vi "Methods_Insert Dividers.vi"(11 "Methods[] In":T1(array[cluster])) -> (3 "Methods[] Out":T1(array[cluster]))   [LabVIEW 2023] (continued)
, "Class Name (unlocalized)"="EventStructure", "Class Name (localized)"="EventStructure"}, "Method Info"={"Unique ID string"="5191803", "Data name"="SetHandledEvents", "Short name (localized)"="SetHandledEvents", "Long name (localized)"="Set Handled Events"}, "Method Flags"={"IsDeprecated"=FALSE, "IsPrivate"=FALSE, "IsScripting"=TRUE, "IsNotInRun-Time"=TRUE}, "Divider"=FALSE}, {"Class Info"={"Unique ID string"="16458", "Parent ID string"="16406", "Class Name (unlocalized)"="EventStructure", "Class Name (localized)"="EventStructure"}, "Method Info"={"Unique ID string"="5191804", "Data name"="GetHandledEventsPriv", "Short name (localized)"="GetHandledEventsPriv", "Long name (localized)"="Get Handled Events (Private)"}, "Method Flags"={"IsDeprecated"=FALSE, "IsPrivate"=TRUE, "IsScripting"=TRUE, "IsNotInRun-Time"=TRUE}, "Divider"=FALSE}, {"Class Info"={"Unique ID string"="16458", "Parent ID string"="16406", "Class Name (unlocalized)"="EventStructure", "Class Name (localized)"="EventStructure"}, "Method Info"={"Unique ID string"="5191805", "Data name"="SetHandledEventsPriv", "Short name (localized)"="SetHandledEventsPriv", "Long name (localized)"="Set Handled Events (Private)"}, "Method Flags"={"IsDeprecated"=FALSE, "IsPrivate"=TRUE, "IsScripting"=TRUE, "IsNotInRun-Time"=TRUE}, "Divider"=FALSE}, {"Class Info"={"Unique ID string"="16459", "Parent ID string"="36", "Class Name (unlocalized)"="FlatSequence", "Class Name (localized)"="FlatSequence"}, "Method Info"={"Unique ID string"="3578b800", "Data name"="Add Frame", "Short name (localized)"="Add Frame", "Long name (localized)"="Add Frame"}, "Method Flags"={"IsDeprecated"=FALSE, "IsPrivate"=FALSE, "IsScripting"=TRUE, "IsNotInRun-Time"=FALSE}, "Divider"=FALSE}, {"Class Info"={"Unique ID string"="16459", "Parent ID string"="36", "Class Name (unlocalized)"="FlatSequence", "Class Name (localized)"="FlatSequence"}, "Method Info"={"Unique ID string"="3578b801", "Data name"="Remove Frame", "Short name (localized)"="Remove Frame", "Long name (localized)"="Remove Frame"}, "Method Flags"={"IsDeprecated"=FALSE, "IsPrivate"=FALSE, "IsScripting"=TRUE, "IsNotInRun-Time"=FALSE}, "Divider"=FALSE}, {"Class Info"={"Unique ID string"="16459", "Parent ID string"="36", "Class Name (unlocalized)"="FlatSequence", "Class Name (localized)"="FlatSequence"}, "Method Info"={"Unique ID string"="3578b802", "Data name"="Auto Size", "Short name (localized)"="Auto Size", "Long name (localized)"="Auto Size"}, "Method Flags"={"IsDeprecated"=FALSE, "IsPrivate"=FALSE, "IsScripting"=TRUE, "IsNotInRun-Time"=FALSE}, "Divider"=FALSE}, {"Class Info"={"Unique ID string"="16459", "Parent ID string"="36", "Class Name (unlocalized)"="FlatSequence", "Class Name (localized)"="FlatSequence"}, "Method Info"={"Unique ID string"="3578b803", "Data name"="Remove Flat Sequence", "Short name (localized)"="Remove Flat Sequence", "Long name (localized)"="Remove Flat Sequence"}, "Method Flags"={"IsDeprecated"=FALSE, "IsPrivate"=FALSE, "IsScripting"=TRUE, "IsNotInRun-Time"=FALSE}, "Divider"=FALSE}, {"Class Info"={"Unique ID string"="16459", "Parent ID string"="36", "Class Name (unlocalized)"="FlatSequence", "Class Name (localized)"="FlatSequence"}, "Method Info"={"Unique ID string"="3578b805", "Data name"="Convert To TimedSequence", "Short name (localized)"="Convert To TimedSequence", "Long name (localized)"="Convert To Timed Sequence"}, "Method Flags"={"IsDeprecated"=FALSE, "IsPrivate"=FALSE, "IsScripting"=TRUE, "IsNotInRun-Time"=FALSE}, "Divider"=FALSE}, {"Class Info"={"Unique ID string"="16463", "Parent ID string"="3", "Class Name (unlocalized)"="SubWizard", "Class Name (localized)"="SubWizard"}, "Method Info"={"Unique ID string"="31942800", "Data name"="LockObject", "Short name (localized)"="LockObject", "Long name (localized)"="Lock Object"}, "Method Flags"={"IsDeprecated"=FALSE, "IsPrivate"=FALSE, "IsScripting"=TRUE, "IsNotInRun-Time"=FALSE}, "Divider"=FALSE}, {"Class Info"={"Unique ID string"="16463", "Parent ID string"="3", "Class Name (unlocalized)"="SubWizard", "Class Name (localized)"="SubWizard"}, "Method Info"={"Unique ID string"="31942801", "Data name"="UnLock Object", "Short name (localized)"="UnLock Object", "Long name (localized)"="Unlock Object"}, "Method Flags"={"IsDeprecated"=FALSE, "IsPrivate"=FALSE, "IsScripting"=TRUE, "IsNotInRun-Time"=FALSE}, "Divider"=FALSE}, {"Class Info"={"Unique ID string"="16463", "Parent ID string"="3", "Class Name (unlocalized)"="SubWizard", "Class Name (localized)"="SubWizard"}, "Method Info"={"Unique ID string"="31942802", "Data name"="Is Locked By Me", "Short name (localized)"="Is Locked By Me", "Long name (localized)"="Is Locked By Me"}, "Method Flags"={"IsDeprecated"=FALSE, "IsPrivate"=FALSE, "IsScripting"=TRUE, "IsNotInRun-Time"=FALSE}, "Divider"=FALSE}, {"Class Info"={"Unique ID string"="16463", "Parent ID string"="3", "Class Name (unlocalized)"="SubWizard", "Class Name (localized)"="SubWizard"}, "Method Info"={"Unique ID string"="31942803", "Data name"="Lock Const", "Short name (localized)"="Lock Const", "Long name (localized)"="Lock Const"}, "Method Flags"={"IsDeprecated"=FALSE, "IsPrivate"=FALSE, "IsScripting"=TRUE, "IsNotInRun-Time"=FALSE}, "Divider"=FALSE}, {"Class Info"={"Unique ID string"="16463", "Parent ID string"="3", "Class Name (unlocalized)"="SubWizard", "Class Name (localized)"="SubWizard"}, "Method Info"={"Unique ID string"="31942804", "Data name"="UnLock Const", "Short name (localized)"="UnLock Const", "Long name (localized)"="Unlock Const"}, "Method Flags"={"IsDeprecated"=FALSE, "IsPrivate"=FALSE, "IsScripting"=TRUE, "IsNotInRun-Time"=FALSE}, "Divider"=FALSE}, {"Class Info"={"Unique ID string"="16467", "Parent ID string"="16435", "Class Name (unlocalized)"="TimedLoop", "Class Name (localized)"="TimedLoop"}, "Method Info"={"Unique ID string"="5afcf000", "Data name"="Replace With WhileLoop", "Short name (localized)"="Replace With WhileLoop", "Long name (localized)"="Replace With WhileLoop"}, "Method Flags"={"IsDeprecated"=FALSE, "IsPrivate"=FALSE, "IsScripting"=TRUE, "IsNotInRun-Time"=FALSE}, "Divider"=FALSE}, {"Class Info"={"Unique ID string"="16467", "Parent ID string"="16435", "Class Name (unlocalized)"="TimedLoop", "Class Name (localized)"="TimedLoop"}, "Method Info"={"Unique ID string"="5afcf001", "Data name"="Replace With TimedSeq", "Short name (localized)"="Replace With TimedSeq", "Long name (localized)"="Replace With TimedSequence"}, "Method Flags"={"IsDeprecated"=FALSE, "IsPrivate"=FALSE, "IsScripting"=TRUE, "IsNotInRun-Time"=FALSE}, "Divider"=FALSE}, {"Class Info"={"Unique ID string"="16472", "Parent ID string"="16384", "Class Name (unlocalized)"="SimDiagram", "Class Name (localized)"="SimDiagram"}, "Method Info"={"Unique ID string"="790ac00", "Data name"="CopyToCompanion", "Short name (localized)"="CopyToCompanion", "Long name (localized)"="CopyToCompanion"}, "Method Flags"={"IsDeprecated"=FALSE, "IsPrivate"=TRUE, "IsScripting"=TRUE, "IsNotInRun-Time"=FALSE}, "Divider"=FALSE}, {"Class Info"={"Unique ID string"="16472", "Parent ID string"="16384", "Class Name (unlocalized)"="SimDiagram", "Class Name (localized)"="SimDiagram"}, "Method Info"={"Unique ID string"="790ac01", "Data name"="setNodeMap", "Short name (localized)"="setNodeMap", "Long name (localized)"="setNodeMap"}, "Method Flags"={"IsDeprecated"=FALSE, "IsPrivate"=TRUE, "IsScripting"=TRUE, "IsNotInRun-Time"=FALSE}, "Divider"=FALSE}, {"Class Info"={"Unique ID string"="16472", "Parent ID string"="16384", "Class Name (unlocalized)"="SimDiagram", "Class Name (localized)"="SimDiagram"}, "Method Info"={"Unique ID string"="790ac02", "Data name"="setSignalMap", "Short name (localized)"="setSignalMap", "Long name (localized)"="setSignalMap"}, "Method Flags"={"IsDeprecated"=FALSE, "IsPrivate"=TRUE, "IsScripting"=TRUE, "IsNotInRun-Time"=FALSE}, "Divider"=FALSE}, {"Class Info"={"Unique ID string"="16472", "Parent ID string"="16384", "Class Name (unlocalized)"="SimDiagram", "Class Name (localized)"="SimDiagram"}, "Method Info"={"Unique ID string"="790ac03", "Data name"="SubsystemFromSelection", "Short name (localized)"="SubsystemFromSelection", "Long name (localized)"="Subsystem From Selection"}, "Method Flags"={"IsDeprecated"=FALSE, "IsPrivate"=TRUE, "IsScripting"=TRUE, "IsNotInRun-Time"=FALSE}, "Divider"=FALSE}, {"Class Info"={"Unique ID string"="16473", "Parent ID string"="16384", "Class Name (unlocalized)"="CompanionDiagram", "Class Name (localized)"="CompanionDiagram"}, "Method Info"={"Unique ID string"="7684bc00", "Data name"="SplitCaseStruct", "Short name (localized)"="SplitCaseStruct", "Long name (localized)"="SplitCaseStruct"}, "Method Flags"={"IsDeprecated"=FALSE, "IsPrivate"=TRUE, "IsScripting"=TRUE, "IsNotInRun-Time"=TRUE}, "Divider"=FALSE}, {"Class Info"={"Unique ID string"="16476", "Parent ID string"="16410", "Class Name (unlocalized)"="Bundler", "Class Name (localized)"="Bundler"}, "Method Info"={"Unique ID string"="570ad000", "Data name"="AddInputAfter", "Short name (localized)"="AddInputAfter", "Long name (localized)"="AddInputAfter"}, "Method Flags"={"IsDeprecated"=FALSE, "IsPrivate"=FALSE, "IsScripting"=TRUE, "IsNotInRun-Time"=TRUE}, "Divider"=FALSE}, {"Class Info"={"Unique ID string"="16476", "Parent ID string"="16410", "Class Name (unlocalized)"="Bundler", "Class Name (localized)"="Bundler"}, "Method Info"={"Unique ID string"="570ad001", "Data name"="RemoveInput", "Short name (localized)"="RemoveInput", "Long name (localized)"="RemoveInput"}, "Method Flags"={"IsDeprecated"=FALSE, "IsPrivate"=FALSE, "IsScripting"=TRUE, "IsNotInRun-Time"=TRUE}, "Divider"=FALSE}, {"Class Info"={"Unique ID string"="16477", "Parent ID string"="16410", "Class Name (unlocalized)"="Unbundler", "Class Name (localized)"="Unbundler"}, "Method Info"={"Unique ID string"="5cc5a000", "Data name"="AddOutputAfter", "Short name (localized)"="AddOutputAfter", "Long name (localized)"="Add Output After"}, "Method Flags"={"IsDeprecated"=FALSE, "IsPrivate"=FALSE, "IsScripting"=TRUE, "IsNotInRun-Time"=TRUE}, "Divider"=FALSE}, {"Class Info"={"Unique ID string"="16477", "Parent ID string"="16410", "Class Name (unlocalized)"="Unbundler", "Class Name (localized)"="Unbundler"}, "Method Info"={"Unique ID string"="5cc5a001", "Data name"="RemoveOutput", "Short name (localized)"="RemoveOutput", "Long name (localized)"="Remove Output"}, "Method Flags"={"IsDeprecated"=FALSE, "IsPrivate"=FALSE, "IsScripting"=TRUE, "IsNotInRun-Time"=TRUE}, "Divider"=FALSE}, {"Class Info"={"Unique ID string"="16485", "Parent ID string"="16421", "Class Name (unlocalized)"="XNode", "Class Name (localized)"="XNode"}, "Method Info"={"Unique ID string"="5f11b402", "Data name"="Message", "Short name (localized)"="Message", "Long name (localized)"="Message"}, "Method Flags"={"IsDeprecated"=FALSE, "IsPrivate"=TRUE, "IsScripting"=TRUE, "IsNotInRun-Time"=TRUE}, "Divider"=FALSE}, {"Class Info"={"Unique ID string"="16485", "Parent ID string"="16421", "Class Name (unlocalized)"="XNode", "Class Name (localized)"="XNode"}, "Method Info"={"Unique ID string"="5f11b403", "Data name"="AddLinkerReference", "Short name (localized)"="AddLinkerReference", "Long name (localized)"="AddLinkerReference"}, "Method Flags"={"IsDeprecated"=FALSE, "IsPrivate"=TRUE, "IsScripting"=TRUE, "IsNotInRun-Time"=TRUE}, "Divider"=FALSE}, {"Class Info"={"Unique ID string"="16485", "Parent ID string"="16421", "Class Name (unlocalized)"="XNode", "Class Name (localized)"="XNode"}, "Method Info"={"Unique ID string"="5f11b404", "Data name"="GetLinkerReference", "Short name (localized)"="GetLinkerReference", "Long name (localized)"="GetLinkerReference"}, "Method Flags"={"IsDeprecated"=FALSE, "IsPrivate"=TRUE, "IsScripting"=TRUE, "IsNotInRun-Time"=TRUE}, "Divider"=FALSE}, {"Class Info"={"Unique ID string"="16485", "Parent ID string"="16421", "Class Name (unlocalized)"="XNode", "Class Name (localized)"="XNode"}, "Method Info"={"Unique ID string"="5f11b405", "Data name"="RemoveLinkerReference", "Short name (localized)"="RemoveLinkerReference", "Long name (localized)"="Remove Linker Reference"}, "Method Flags"={"IsDeprecated"=FALSE, "IsPrivate"=TRUE, "IsScripting"=TRUE, "IsNotInRun-Time"=TRUE}, "Divider"=FALSE}, {"Class Info"={"Unique ID string"="16485", "Parent ID string"="16421", "Class Name (unlocalized)"="XNode", "Class Name (localized)"="XNode"}, "Method Info"={"Unique ID string"="5f11b406", "Data name"="RemoveXNode", "Short name (localized)"="RemoveXNode", "Long name (localized)"="Remove XNode"}, "Method Flags"={"IsDeprecated"=FALSE, "IsPrivate"=TRUE, "IsScripting"=TRUE, "IsNotInRun-Time"=FALSE}, "Divider"=FALSE}, {"Class Info"={"Unique ID string"="16485", "Parent ID string"="16421", "Class Name (unlocalized)"="XNode", "Class Name (localized)"="XNode"}, "Method Info"={"Unique ID string"="5f11b407", "Data name"="GetOtherTerminal", "Short name (localized)"="GetOtherTerminal", "Long name (localized)"="Get Other Terminal"}, "Method Flags"={"IsDeprecated"=FALSE, "IsPrivate"=TRUE, "IsScripting"=TRUE, "IsNotInRun-Time"=FALSE}, "Divider"=FALSE}, {"Class Info"={"Unique ID string"="16485", "Parent ID string"="16421", "Class Name (unlocalized)"="XNode", "Class Name (localized)"="XNode"}, "Method Info"={"Unique ID string"="5f11b408", "Data name"="GenerateCode", "Short name (localized)"="GenerateCode", "Long name (localized)"="Generate Code"}, "Method Flags"={"IsDeprecated"=FALSE, "IsPrivate"=TRUE, "IsScripting"=TRUE, "IsNotInRun-Time"=TRUE}, "Divider"=FALSE}, {"Class Info"={"Unique ID string"="16485", "Parent ID string"="16421", "Class Name (unlocalized)"="XNode", "Class Name (localized)"="XNode"}, "Method Info"={"Unique ID string"="5f11b40a", "Data name"="GetTermByID", "Short name (localized)"="GetTermByID", "Long name (localized)"="Get Term By ID"}, "Method Flags"={"IsDeprecated"=FALSE, "IsPrivate"=TRUE, "IsScripting"=TRUE, "IsNotInRun-Time"=FALSE}, "Divider"=FALSE}, {"Class Info"={"Unique ID string"="16485", "Parent ID string"="16421", "Class Name (unlocalized)"="XNode", "Class Name (localized)"="XNode"}, "Method Info"={"Unique ID string"="5f11b40b", "Data name"="XSFP.Set Terms", "Short name (localized)"="XSFP.Set Terms", "Long name (localized)"="XSFP:Set Terminals"}, "Method Flags"={"IsDeprecated"=FALSE, "IsPrivate"=TRUE, "IsScripting"=TRUE, "IsNotInRun-Time"=FALSE}, "Divider"=FALSE}, {"Class Info"={"Unique ID string"="16485", "Parent ID string"="16421", "Class Name (unlocalized)"="XNode", "Class Name (localized)"="XNode"}, "Method Info"={"Unique ID string"="5f11b40c", "Data name"="XSFP.SetBounds", "Short name (localized)"="XSFP.SetBounds", "Long name (localized)"="XSFP:Set Bounds"}, "Method Flags"={"IsDeprecated"=FALSE, "IsPrivate"=TRUE, "IsScripting"=TRUE, "IsNotInRun-Time"=FALSE}, "Divider"=FALSE}, {"Class Info"={"Unique ID string"="16485", "Parent ID string"="16421", "Class Name (unlocalized)"="XNode", "Class Name (localized)"="XNode"}, "Method Info"={"Unique ID string"="5f11b40d", "Data name"="SelectMenuNoReply", "Short name (localized)"="SelectMenuNoReply", "Long name (localized)"="SelectMenu No Reply"}, "Method Flags"={"IsDeprecated"=FALSE, "IsPrivate"=TRUE, "IsScripting"=TRUE, "IsNotInRun-Time"=FALSE}, "Divider"=FALSE}, {"Class Info"={"Unique ID string"="16485", "Parent ID string"="16421", "Class Name (unlocalized)"="XNode", "Class Name (localized)"="XNode"}, "Method Info"={"Unique ID string"="5f11b40e", "Data name"="ValueForTerm", "Short name (localized)"="ValueForTerm", "Long name (localized)"="ValueForTerm"}, "Method Flags"={"IsDeprecated"=FALSE, "IsPrivate"=TRUE, "IsScripting"=TRUE, "IsNotInRun-Time"=TRUE}, "Divider"=FALSE}, {"Class Info"={"Unique ID string"="16485", "Parent ID string"="16421", "Class Name (unlocalized)"="XNode", "Class Name (localized)"="XNode"}, "Method Info"={"Unique ID string"="5f11b40f", "Data name"="XSFP.Clear Diagram", "Short name (localized)"="XSFP.Clear Diagram", "Long name (localized)"="XSFP:Clear"}, "Method Flags"={"IsDeprecated"=FALSE, "IsPrivate"=TRUE, "IsScripting"=TRUE, "IsNotInRun-Time"=FALSE}, "Divider"=FALSE}, {"Class Info"={"Unique ID string"="16487", "Parent ID string"="16406", "Class Name (unlocalized)"="DisableStructure", "Class Name (localized)"="DisableStructure"}, "Method Info"={"Unique ID string"="669be000", "Data name"="Get Frame Index", "Short name (localized)"="Get Frame Index", "Long name (localized)"="Get Frame Index"}, "Method Flags"={"IsDeprecated"=FALSE, "IsPrivate"=FALSE, "IsScripting"=TRUE, "IsNotInRun-Time"=FALSE}, "Divider"=FALSE}, {"Class Info"={"Unique ID string"="16487", "Parent ID string"="16406", "Class Name (unlocalized)"="DisableStructure", "Class Name (localized)"="DisableStructure"}, "Method Info"={"Unique ID string"="669be001", "Data name"="Remove Empty Frames", "Short name (localized)"="Remove Empty Frames", "Long name (localized)"="Remove Empty Frames"}, "Method Flags"={"IsDeprecated"=FALSE, "IsPrivate"=FALSE, "IsScripting"=TRUE, "IsNotInRun-Time"=FALSE}, "Divider"=FALSE}, {"Class Info"={"Unique ID string"="16487", "Parent ID string"="16406", "Class Name (unlocalized)"="DisableStructure", "Class Name (localized)"="DisableStructure"}, "Method Info"={"Unique ID string"="669be002", "Data name"="Change Disable Style", "Short name (localized)"="Change Disable Style", "Long name (localized)"="Change Disable Style"}, "Method Flags"={"IsDeprecated"=FALSE, "IsPrivate"=FALSE, "IsScripting"=TRUE, "IsNotInRun-Time"=FALSE}, "Divider"=FALSE}, {"Class Info"={"Unique ID string"="16488", "Parent ID string"="16384", "Class Name (unlocalized)"="SDFDiagram", "Class Name (localized)"="SDFDiagram"}, "Method Info"={"Unique ID string"="f6a0400", "Data name"="CopyToSDFCompanion", "Short name (localized)"="CopyToSDFCompanion", "Long name (localized)"="Copy To SDF Companion"}, "Method Flags"={"IsDeprecated"=FALSE, "IsPrivate"=TRUE, "IsScripting"=TRUE, "IsNotInRun-Time"=FALSE}, "Divider"=FALSE}, {"Class Info"={"Unique ID string"="16495", "Parent ID string"="16459", "Class Name (unlocalized)"="TimeFlatSequence", "Class Name (localized)"="TimeFlatSequence"}, "Method Info"={"Unique ID string"="51167400", "Data name"="Add Frame", "Short name (localized)"="Add Frame", "Long name (localized)"="Add Frame (not implemented)"}, "Method Flags"={"IsDeprecated"=FALSE, "IsPrivate"=TRUE, "IsScripting"=TRUE, "IsNotInRun-Time"=FALSE}, "Divider"=FALSE}, {"Class Info"={"Unique ID string"="16496", "Parent ID string"="16404", "Class Name (unlocalized)"="TimedSequence", "Class Name (localized)"="TimedSequence"}, "Method Info"={"Unique ID string"="6c4f3800", "Data name"="Convert To FlatSeq", "Short name (localized)"="Convert To FlatSeq", "Long name (localized)"="Convert To FlatSequence"}, "Method Flags"={"IsDeprecated"=FALSE, "IsPrivate"=FALSE, "IsScripting"=TRUE, "IsNotInRun-Time"=FALSE}, "Divider"=FALSE}, {"Class Info"={"Unique ID string"="16496", "Parent ID string"="16404", "Class Name (unlocalized)"="TimedSequence", "Class Name (localized)"="TimedSequence"}, "Method Info"={"Unique ID string"="6c4f3801", "Data name"="Convert T oTimedLoop", "Short name (localized)"="Convert T oTimedLoop", "Long name (localized)"="Convert To TimedLoop"}, "Method Flags"={"IsDeprecated"=FALSE, "IsPrivate"=FALSE, "IsScripting"=TRUE, "IsNotInRun-Time"=FALSE}, "Divider"=FALSE}, {"Class Info"={"Unique ID string"="16499", "Parent ID string"="16409", "Class Name (unlocalized)"="MathScriptNode", "Class Name (localized)"="MathScriptNode"}, "Method Info"={"Unique ID string"="336cd800", "Data name"="ConfigUserFunc", "Short name (localized)"="ConfigUserFunc", "Long name (localized)"="Configure User Function"}, "Method Flags"={"IsDeprecated"=FALSE, "IsPrivate"=TRUE, "IsScripting"=TRUE, "IsNotInRun-Time"=TRUE}, "Divider"=FALSE}, {"Class Info"={"Unique ID string"="16499", "Parent ID string"="16409", "Class Name (unlocalized)"="MathScriptNode", "Class Name (localized)"="MathScriptNode"}, "Method Info"={"Unique ID string"="336cd801", "Data name"="AttachMSNProbe", "Short name (localized)"="AttachMSNProbe", "Long name (localized)"="Attach MathScript Probe"}, "Method Flags"={"IsDeprecated"=FALSE, "IsPrivate"=TRUE, "IsScripting"=TRUE, "IsNotInRun-Time"=FALSE}, "Divider"=FALSE}, {"Class Info"={"Unique ID string"="16499", "Parent ID string"="16409", "Class Name (unlocalized)"="MathScriptNode", "Class Name (localized)"="MathScriptNode"}, "Method Info"={"Unique ID string"="336cd802", "Data name"="SetMSNBPOnLine", "Short name (localized)"="SetMSNBPOnLine", "Long name (localized)"="Set MathScript Node Line Breakpoint"}, "Method Flags"={"IsDeprecated"=FALSE, "IsPrivate"=FALSE, "IsScripting"=TRUE, "IsNotInRun-Time"=FALSE}, "Divider"=FALSE}, {"Class Info"={"Unique ID string"="16499", "Parent ID string"="16409", "Class Name (unlocalized)"="MathScriptNode", "Class Name (localized)"="MathScriptNode"}, "Method Info"={"Unique ID string"="336cd803", "Data name"="ClearFBoxLineNodes", "Short name (localized)"="ClearFBoxLineNodes", "Long name (localized)"="Clear FBoxLine Stored Nodes"}, "Method Flags"={"IsDeprecated"=FALSE, "IsPrivate"=TRUE, "IsScripting"=TRUE, "IsNotInRun-Time"=FALSE}, "Divider"=FALSE}, {"Class Info"={"Unique ID string"="16499", "Parent ID string"="16409", "Class Name (unlocalized)"="MathScriptNode", "Class Name (localized)"="MathScriptNode"}, "Method Info"={"Unique ID string"="336cd804", "Data name"="NeedsGPropTypes", "Short name (localized)"="NeedsGPropTypes", "Long name (localized)"="NeedsGPropTypes"}, "Method Flags"={"IsDeprecated"=FALSE, "IsPrivate"=TRUE, "IsScripting"=TRUE, "IsNotInRun-Time"=FALSE}, "Divider"=FALSE}, {"Class Info"={"Unique ID string"="16503", "Parent ID string"="36", "Class Name (unlocalized)"="AbstractDiagram", "Class Name (localized)"="AbstractDiagram"}, "Method Info"={"Unique ID string"="6375400", "Data name"="Paste", "Short name (localized)"="Paste", "Long name (localized)"="Paste"}, "Method Flags"={"IsDeprecated"=FALSE, "IsPrivate"=FALSE, "IsScripting"=TRUE, "IsNotInRun-Time"=TRUE}, "Divider"=FALSE}, {"Class Info"={"Unique ID string"="16503", "Parent ID string"="36", "Class Name (unlocalized)"="AbstractDiagram", "Class Name (localized)"="AbstractDiagram"}, "Method Info"={"Unique ID string"="6375401", "Data name"="Select All", "Short name (localized)"="Select All", "Long name (localized)"="Select All"}, "Method Flags"={"IsDeprecated"=FALSE, "IsPrivate"=FALSE, "IsScripting"=TRUE, "IsNotInRun-Time"=TRUE}, "Divider"=FALSE}, {"Class Info"={"Unique ID string"="16503", "Parent ID string"="36", "Class Name (unlocalized)"="AbstractDiagram", "Class Name (localized)"="AbstractDiagram"}, "Method Info"={"Unique ID string"="6375402", "Data name"="MakeSpace", "Short name (localized)"="MakeSpace", "Long name (localized)"="Make Space"}, "Method Flags"={"IsDeprecated"=FALSE, "IsPrivate"=FALSE, "IsScripting"=TRUE, "IsNotInRun-Time"=FALSE}, "Divider"=FALSE}, {"Class Info"={"Unique ID string"="16503", "Parent ID string"="36", "Class Name (unlocalized)"="AbstractDiagram", "Class Name (localized)"="AbstractDiagram"}, "Method Info"={"Unique ID string"="6375403", "Data name"="Shrink Wrap Structs", "Short name (localized)"="Shrink Wrap Structs", "Long name (localized)"="Shrink Wrap Structures"}, "Method Flags"={"IsDeprecated"=FALSE, "IsPrivate"=FALSE, "IsScripting"=TRUE, "IsNotInRun-Time"=FALSE}, "Divider"=FALSE}, {"Class Info"={"Unique ID string"="16503", "Parent ID string"="36", "Class Name (unlocalized)"="AbstractDiagram", "Class Name (localized)"="AbstractDiagram"}, "Method Info"={"Unique ID string"="6375404", "Data name"="Gen Script Diagram", "Short name (localized)"="Gen Script Diagram", "Long name (localized)"="Gen Script Diagram"}, "Method Flags"={"IsDeprecated"=FALSE, "IsPrivate"=TRUE, "IsScripting"=TRUE, "IsNotInRun-Time"=TRUE}, "Divider"=FALSE}, {"Class Info"={"Unique ID string"="16503", "Parent ID string"="36", "Class Name (unlocalized)"="AbstractDiagram", "Class Name (localized)"="AbstractDiagram"}, "Method Info"={"Unique ID string"="6375405", "Data name"="SubVI From Selection", "Short name (localized)"="SubVI From Selection", "Long name (localized)"="SubVI From Selection"}, "Method Flags"={"IsDeprecated"=FALSE, "IsPrivate"=TRUE, "IsScripting"=TRUE, "IsNotInRun-Time"=FALSE}, "Divider"=FALSE}, {"Class Info"={"Unique ID string"="16503", "Parent ID string"="36", "Class Name (unlocalized)"="AbstractDiagram", "Class Name (localized)"="AbstractDiagram"}, "Method Info"={"Unique ID string"="6375406", "Data name"="GetCodeWizRef", "Short name (localized)"="GetCodeWizRef", "Long name (localized)"="Get CodeWizRef"}, "Method Flags"={"IsDeprecated"=FALSE, "IsPrivate"=TRUE, "IsScripting"=TRUE, "IsNotInRun-Time"=TRUE}, "Divider"=FALSE}, {"Class Info"={"Unique ID string"="16503", "Parent ID string"="36", "Class Name (unlocalized)"="AbstractDiagram", "Class Name (localized)"="AbstractDiagram"}, "Method Info"={"Unique ID string"="6375407", "Data name"="Create Constant", "Short name (localized)"="Create Constant", "Long name (localized)"="Create Constant From Data Type"}, "Method Flags"={"IsDeprecated"=FALSE, "IsPrivate"=TRUE, "IsScripting"=TRUE, "IsNotInRun-Time"=TRUE}, "Divider"=FALSE}, {"Class Info"={"Unique ID string"="16503", "Parent ID string"="36", "Class Name (unlocalized)"="AbstractDiagram", "Class Name (localized)"="AbstractDiagram"}, "Method Info"={"Unique ID string"="6375408", "Data name"="BuildIGL", "Short name (localized)"="BuildIGL", "Long name (localized)"="Build IGL"}, "Method Flags"={"IsDeprecated"=FALSE, "IsPrivate"=TRUE, "IsScripting"=TRUE, "IsNotInRun-Time"=TRUE}, "Divider"=FALSE}, {"Class Info"={"Unique ID string"="16503", "Parent ID string"="36", "Class Name (unlocalized)"="AbstractDiagram", "Class Name (localized)"="AbstractDiagram"}, "Method Info"={"Unique ID string"="6375409", "Data name"="RemWireLooseEnds", "Short name (localized)"="RemWireLooseEnds", "Long name (localized)"="Remove Wire Loose Ends"}, "Method Flags"={"IsDeprecated"=FALSE, "IsPrivate"=FALSE, "IsScripting"=TRUE, "IsNotInRun-Time"=TRUE}, "Divider"=FALSE}, {"Class Info"={"Unique ID string"="16512", "Parent ID string"="16421", "Class Name (unlocalized)"="SharedVariableNode", "Class Name (localized)"="SharedVariableNode"}, "Method Info"={"Unique ID string"="55d4ac00", "Data name"="Change to Control", "Short name (localized)"="Change to Control", "Long name (localized)"="Change to Control"}, "Method Flags"={"IsDeprecated"=FALSE, "IsPrivate"=FALSE, "IsScripting"=TRUE, "IsNotInRun-Time"=TRUE}, "Divider"=FALSE}, {"Class Info"={"Unique ID string"="16512", "Parent ID string"="16421", "Class Name (unlocalized)"="SharedVariableNode", "Class Name (localized)"="SharedVariableNode"}, "Method Info"={"Unique ID string"="55d4ac01", "Data name"="Change to Indicator", "Short name (localized)"="Change to Indicator", "Long name (localized)"="Change to Indicator"}, "Method Flags"={"IsDeprecated"=FALSE, "IsPrivate"=FALSE, "IsScripting"=TRUE, "IsNotInRun-Time"=TRUE}, "Divider"=FALSE}, {"Class Info"={"Unique ID string"="16512", "Parent ID string"="16421", "Class Name (unlocalized)"="SharedVariableNode", "Class Name (localized)"="SharedVariableNode"}, "Method Info"={"Unique ID string"="55d4ac02", "Data name"="Change to Constant", "Short name (localized)"="Change to Constant", "Long name (localized)"="Change to Constant"}, "Method Flags"={"IsDeprecated"=FALSE, "IsPrivate"=FALSE, "IsScripting"=TRUE, "IsNotInRun-Time"=TRUE}, "Divider"=FALSE}, {"Class Info"={"Unique ID string"="16512", "Parent ID string"="16421", "Class Name (unlocalized)"="SharedVariableNode", "Class Name (localized)"="SharedVariableNode"}, "Method Info"={"Unique ID string"="55d4ac03", "Data name"="CopyLinkageFromVarXNode", "Short name (localized)"="CopyLinkageFromVarXNode", "Long name (localized)"="Copy Linkage From VarXNode"}, "Method Flags"={"IsDeprecated"=FALSE, "IsPrivate"=TRUE, "IsScripting"=TRUE, "IsNotInRun-Time"=TRUE}, "Divider"=FALSE}, {"Class Info"={"Unique ID string"="16512", "Parent ID string"="16421", "Class Name (unlocalized)"="SharedVariableNode", "Class Name (localized)"="SharedVariableNode"}, "Method Info"={"Unique ID string"="55d4ac04", "Data name"="MarkVIRelative", "Short name (localized)"="MarkVIRelative", "Long name (localized)"="MarkVIRelative"}, "Method Flags"={"IsDeprecated"=FALSE, "IsPrivate"=TRUE, "IsScripting"=TRUE, "IsNotInRun-Time"=TRUE}, "Divider"=FALSE}, {"Class Info"={"Unique ID string"="16516", "Parent ID string"="16404", "Class Name (unlocalized)"="InPlaceElementStructure", "Class Name (localized)"="InPlaceElementStructure"}, "Method Info"={"Unique ID string"="658ea800", "Data name"="Add In Place Pair", "Short name (localized)"="Add In Place Pair", "Long name (localized)"="Add In Place Pair"}, "Method Flags"={"IsDeprecated"=FALSE, "IsPrivate"=FALSE, "IsScripting"=TRUE, "IsNotInRun-Time"=TRUE}, "Divider"=FALSE}, {"Class Info"={"Unique ID string"="16518", "Parent ID string"="16517", "Class Name (unlocalized)"="InPlaceArrayNode", "Class Name (localized)"="InPlaceArrayNode"}, "Method Info"={"Unique ID string"="1614ec00", "Data name"="Resize", "Short name (localized)"="Resize", "Long name (localized)"="Resize"}, "Method Flags"={"IsDeprecated"=FALSE, "IsPrivate"=FALSE, "IsScripting"=TRUE, "IsNotInRun-Time"=TRUE}, "Divider"=FALSE}, {"Class Info"={"Unique ID string"="16519", "Parent ID string"="16517", "Class Name (unlocalized)"="InPlaceClusterNode", "Class Name (localized)"="InPlaceClusterNode"}, "Method Info"={"Unique ID string"="7616e400", "Data name"="Resize", "Short name (localized)"="Resize", "Long name (localized)"="Resize"}, "Method Flags"={"IsDeprecated"=FALSE, "IsPrivate"=FALSE, "IsScripting"=TRUE, "IsNotInRun-Time"=TRUE}, "Divider"=FALSE}, {"Class Info"={"Unique ID string"="16519", "Parent ID string"="16517", "Class Name (unlocalized)"="InPlaceClusterNode", "Class Name (localized)"="InPlaceClusterNode"}, "Method Info"={"Unique ID string"="7616e401", "Data name"="AddOutputAfter", "Short name (localized)"="AddOutputAfter", "Long name (localized)"="Add Output After"}, "Method Flags"={"IsDeprecated"=FALSE, "IsPrivate"=FALSE, "IsScripting"=TRUE, "IsNotInRun-Time"=TRUE}, "Divider"=FALSE}, {"Class Info"={"Unique ID string"="16519", "Parent ID string"="16517", "Class Name (unlocalized)"="InPlaceClusterNode", "Class Name (localized)"="InPlaceClusterNode"}, "Method Info"={"Unique ID string"="7616e402", "Data name"="RemoveOutput", "Short name (localized)"="RemoveOutput", "Long name (localized)"="Remove Output"}, "Method Flags"={"IsDeprecated"=FALSE, "IsPrivate"=FALSE, "IsScripting"=TRUE, "IsNotInRun-Time"=TRUE}, "Divider"=FALSE}, {"Class Info"={"Unique ID string"="16522", "Parent ID string"="16421", "Class Name (unlocalized)"="FeedbackNode", "Class Name (localized)"="FeedbackNode"}, "Method Info"={"Unique ID string"="778ed000", "Data name"="RepWithShiftReg", "Short name (localized)"="RepWithShiftReg", "Long name (localized)"="Replace With Shift Register"}, "Method Flags"={"IsDeprecated"=FALSE, "IsPrivate"=FALSE, "IsScripting"=TRUE, "IsNotInRun-Time"=TRUE}, "Divider"=FALSE}, {"Class Info"={"Unique ID string"="16522", "Parent ID string"="16421", "Class Name (unlocalized)"="FeedbackNode", "Class Name (localized)"="FeedbackNode"}, "Method Info"={"Unique ID string"="778ed001", "Data name"="HighlightInit", "Short name (localized)"="HighlightInit", "Long name (localized)"="Highlight Initializer"}, "Method Flags"={"IsDeprecated"=FALSE, "IsPrivate"=FALSE, "IsScripting"=TRUE, "IsNotInRun-Time"=TRUE}, "Divider"=FALSE}, {"Class Info"={"Unique ID string"="16523", "Parent ID string"="16421", "Class Name (unlocalized)"="MathScriptCallByRef", "Class Name (localized)"="MathScriptCallByRef"}, "Method Info"={"Unique ID string"="25021400", "Data name"="Configure", "Short name (localized)"="Configure", "Long name (localized)"="Configure"}, "Method Flags"={"IsDeprecated"=FALSE, "IsPrivate"=TRUE, "IsScripting"=TRUE, "IsNotInRun-Time"=FALSE}, "Divider"=FALSE}, {"Class Info"={"Unique ID string"="16525", "Parent ID string"="16426", "Class Name (unlocalized)"="ConditionalTunnel", "Class Name (localized)"="ConditionalTunnel"}, "Method Info"={"Unique ID string"="5d251800", "Data name"="LinkTun", "Short name (localized)"="LinkTun", "Long name (localized)"="Link Input Tunnel"}, "Method Flags"={"IsDeprecated"=FALSE, "IsPrivate"=FALSE, "IsScripting"=TRUE, "IsNotInRun-Time"=FALSE}, "Divider"=FALSE}, {"Class Info"={"Unique ID string"="16525", "Parent ID string"="16426", "Class Name (unlocalized)"="ConditionalTunnel", "Class Name (localized)"="ConditionalTunnel"}, "Method Info"={"Unique ID string"="5d251801", "Data name"="ClearLinkTun", "Short name (localized)"="ClearLinkTun", "Long name (localized)"="Clear Linked Input Tunnel"}, "Method Flags"={"IsDeprecated"=FALSE, "IsPrivate"=FALSE, "IsScripting"=TRUE, "IsNotInRun-Time"=FALSE}, "Divider"=FALSE}, {"Class Info"={"Unique ID string"="16525", "Parent ID string"="16426", "Class Name (unlocalized)"="ConditionalTunnel", "Class Name (localized)"="ConditionalTunnel"}, "Method Info"={"Unique ID string"="5d251802", "Data name"="LinkTunAndWire", "Short name (localized)"="LinkTunAndWire", "Long name (localized)"="Link Input Tunnel And Wire"}, "Method Flags"={"IsDeprecated"=FALSE, "IsPrivate"=FALSE, "IsScripting"=TRUE, "IsNotInRun-Time"=FALSE}, "Divider"=FALSE}, {"Class Info"={"Unique ID string"="16525", "Parent ID string"="16426", "Class Name (unlocalized)"="ConditionalTunnel", "Class Name (localized)"="ConditionalTunnel"}, "Method Info"={"Unique ID string"="5d251803", "Data name"="RepWithCaseSel", "Short name (localized)"="RepWithCaseSel", "Long name (localized)"="Replace With Case Selector"}, "Method Flags"={"IsDeprecated"=FALSE, "IsPrivate"=FALSE, "IsScripting"=TRUE, "IsNotInRun-Time"=FALSE}, "Divider"=FALSE}, {"Class Info"={"Unique ID string"="16536", "Parent ID string"="16426", "Class Name (unlocalized)"="RegionTunnel", "Class Name (localized)"="RegionTunnel"}, "Method Info"={"Unique ID string"="51af2c00", "Data name"="Unlock", "Short name (localized)"="Unlock", "Long name (localized)"="Unlock"}, "Method Flags"={"IsDeprecated"=FALSE, "IsPrivate"=TRUE, "IsScripting"=TRUE, "IsNotInRun-Time"=TRUE}, "Divider"=FALSE}, {"Class Info"={"Unique ID string"="16537", "Parent ID string"="16404", "Class Name (unlocalized)"="StatechartStructureNode", "Class Name (localized)"="StatechartStructureNode"}, "Method Info"={"Unique ID string"="24fc6000", "Data name"="Create Tunnel(In) Lock", "Short name (localized)"="Create Tunnel(In) Lock", "Long name (localized)"="Create Incoming Tunnel And Lock"}, "Method Flags"={"IsDeprecated"=FALSE, "IsPrivate"=TRUE, "IsScripting"=TRUE, "IsNotInRun-Time"=TRUE}, "Divider"=FALSE}, {"Class Info"={"Unique ID string"="16537", "Parent ID string"="16404", "Class Name (unlocalized)"="StatechartStructureNode", "Class Name (localized)"="StatechartStructureNode"}, "Method Info"={"Unique ID string"="24fc6001", "Data name"="Create Tunnel(Out) Lock", "Short name (localized)"="Create Tunnel(Out) Lock", "Long name (localized)"="Create Outgoing Tunnel And Lock"}, "Method Flags"={"IsDeprecated"=FALSE, "IsPrivate"=TRUE, "IsScripting"=TRUE, "IsNotInRun-Time"=TRUE}, "Divider"=FALSE}, {"Class Info"={"Unique ID string"="16543", "Parent ID string"="16406", "Class Name (unlocalized)"="TargetStructureNode", "Class Name (localized)"="TargetStructureNode"}, "Method Info"={"Unique ID string"="45750400", "Data name"="Remove Frame", "Short name (localized)"="Remove Frame", "Long name (localized)"="Remove Frame"}, "Method Flags"={"IsDeprecated"=FALSE, "IsPrivate"=FALSE, "IsScripting"=TRUE, "IsNotInRun-Time"=FALSE}, "Divider"=FALSE}, {"Class Info"={"Unique ID string"="16543", "Parent ID string"="16406", "Class Name (unlocalized)"="TargetStructureNode", "Class Name (localized)"="TargetStructureNode"}, "Method Info"={"Unique ID string"="45750401", "Data name"="Add Frame", "Short name (localized)"="Add Frame", "Long name (localized)"="Add Frame"}, "Method Flags"={"IsDeprecated"=FALSE, "IsPrivate"=FALSE, "IsScripting"=TRUE, "IsNotInRun-Time"=FALSE}, "Divider"=FALSE}, {"Class Info"={"Unique ID string"="16544", "Parent ID string"="16517", "Class Name (unlocalized)"="InPlaceVariantAttributeNode", "Class Name (localized)"="InPlaceVariantAttributeNode"}, "Method Info"={"Unique ID string"="1a44f000", "Data name"="Resize", "Short name (localized)"="Resize", "Long name (localized)"="Resize"}, "Method Flags"={"IsDeprecated"=FALSE, "IsPrivate"=FALSE, "IsScripting"=TRUE, "IsNotInRun-Time"=FALSE}, "Divider"=FALSE}, {"Class Info"={"Unique ID string"="16547", "Parent ID string"="16463", "Class Name (unlocalized)"="ExternalEditorWizard", "Class Name (localized)"="ExternalEditorWizard"}, "Method Info"={"Unique ID string"="1c2e9800", "Data name"="LaunchEd", "Short name (localized)"="LaunchEd", "Long name (localized)"="LaunchEditor"}, "Method Flags"={"IsDeprecated"=FALSE, "IsPrivate"=FALSE, "IsScripting"=TRUE, "IsNotInRun-Time"=TRUE}, "Divider"=FALSE}, {"Class Info"={"Unique ID string"="16548", "Parent ID string"="16517", "Class Name (unlocalized)"="InPlaceMapNode", "Class Name (localized)"="InPlaceMapNode"}, "Method Info"={"Unique ID string"="13c9f800", "Data name"="SetNumKeyValuePairs", "Short name (localized)"="SetNumKeyValuePairs", "Long name (localized)"="Set number of Key/Value Pairs"}, "Method Flags"={"IsDeprecated"=FALSE, "IsPrivate"=FALSE, "IsScripting"=TRUE, "IsNotInRun-Time"=FALSE}, "Divider"=FALSE}, {"Class Info"={"Unique ID string"="16552", "Parent ID string"="16386", "Class Name (unlocalized)"="SetConstant", "Class Name (localized)"="SetConstant"}, "Method Info"={"Unique ID string"="99fb400", "Data name"="ScrollToElement", "Short name (localized)"="ScrollToElement", "Long name (localized)"="Scroll To Element"}, "Method Flags"={"IsDeprecated"=FALSE, "IsPrivate"=FALSE, "IsScripting"=TRUE, "IsNotInRun-Time"=FALSE}, "Divider"=FALSE}, {"Class Info"={"Unique ID string"="16553", "Parent ID string"="16386", "Class Name (unlocalized)"="MapConstant", "Class Name (localized)"="MapConstant"}, "Method Info"={"Unique ID string"="12558400", "Data name"="ScrollToKey", "Short name (localized)"="ScrollToKey", "Long name (localized)"="Scroll To Key"}, "Method Flags"={"IsDeprecated"=FALSE, "IsPrivate"=FALSE, "IsScripting"=TRUE, "IsNotInRun-Time"=FALSE}, "Divider"=FALSE}])   [LabVIEW 2023]
doc: "Insert Divider Element between each major class type. This is used for display and also for reversing the class order in the BundleMagoc dialog.\n\nThis must come before dotted properties are inserted."
panel:
  out "Divider Ct":i32
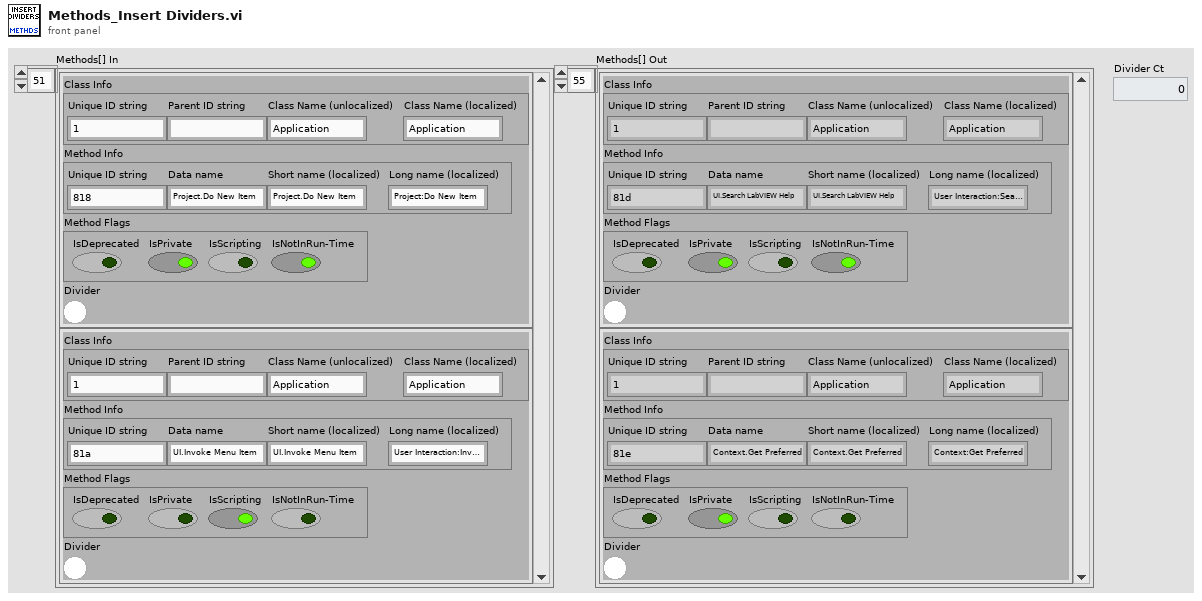
[diagram p1: front panel]
types:
  T1 = cluster{"Class Info":cluster{"Unique ID string":string, "Parent ID string":string, "Class Name (unlocalized)":string, "Class Name (localized)":string}, "Method Info":cluster{"Unique ID string":string, "Data name":string, "Short name (localized)":string, "Long name (localized)":string}, "Method Flags":cluster{"IsDeprecated":bool, "IsPrivate":bool, "IsScripting":bool, "IsNotInRun-Time":bool}, "Divider":bool}[]
  T2 = cluster{"Class Info":cluster{"Unique ID string":string, "Parent ID string":string, "Class Name (unlocalized)":string, "Class Name (localized)":string}, "Method Info":cluster{"Unique ID string":string, "Data name":string, "Short name (localized)":string, "Long name (localized)":string}, "Method Flags":cluster{"IsDeprecated":bool, "IsPrivate":bool, "IsScripting":bool, "IsNotInRun-Time":bool}, "Divider":bool}
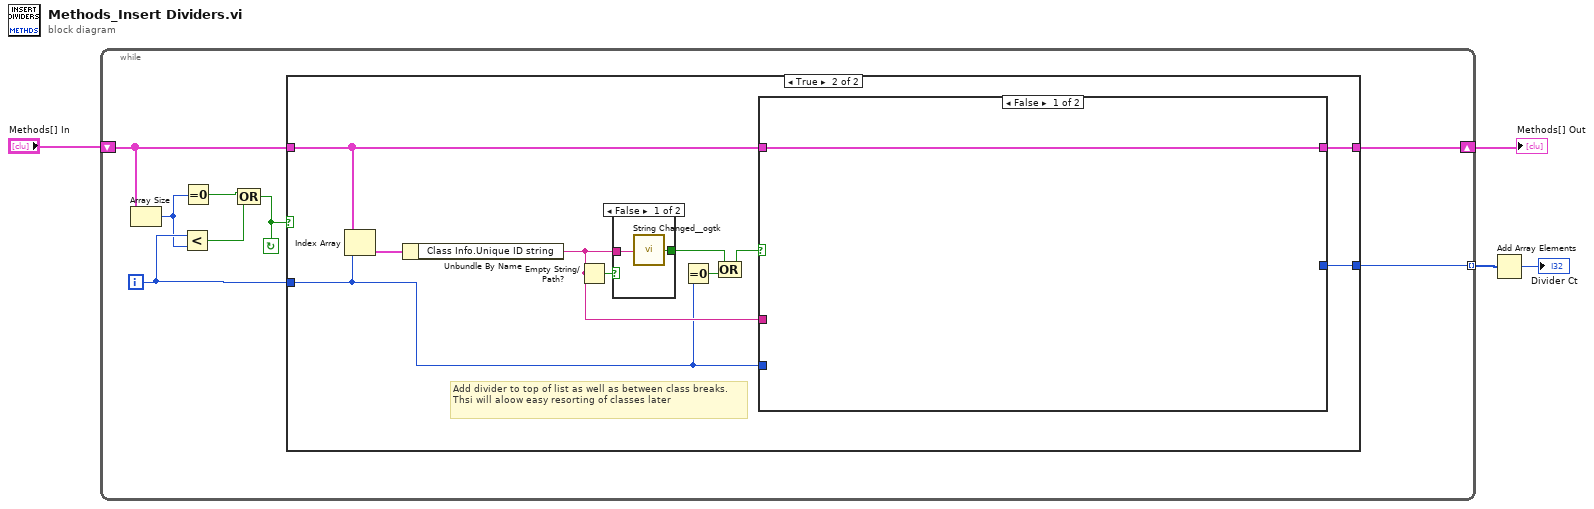
[diagram p0: block diagram]
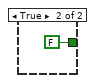
[diagram p3: hidden frame]
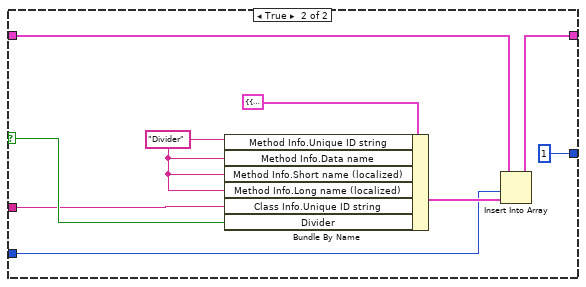
[diagram p4: hidden frame]
diagram:
  n1 = while {
    shift-right: [w10] -> w2
    shift-left: "Methods[] In" -> [w12]
    tunnel: [w11] -> w4 mode=indexing
    i -> [w6]
    stop <- w7 continue-if-true
    n2 = Array Size(array=w12) -> (size(s)=w5:i32)
    n3 = Less?(x=w6, y=w5) -> (x < y?=w8:bool)
    n4 = Equal To 0?(x=w5) -> (x = 0?=w9:bool)
    n5 = Compound Arithmetic op=OR(w9, w8) -> (w7:bool)
    n6 = case shown="True" w7 {
      tunnel: [w13 w23] -> w10
      tunnel: w12 -> [w13 w22]
      tunnel: w6 -> [_ w17]
      tunnel: [_ w21] -> w11
      frame False {
      }
      frame True {
        # "Add divider to top of list as well as between class breaks. Thsi will aloow easy resorting of classes later"
        n7 = Index Array(array=w22, index=w17) -> (element=w19:T2)
        n8 = Unbundle By Name(w19) -> ("Class Info.Unique ID string"=w18:string)
        n9 = Empty String/Path?(string/path=w18) -> (empty?=w20:bool)
        n10 = case shown="False" w20 {
          tunnel: w18 -> [w25 _]
          tunnel: [w24 FALSE ("Changed")] -> w15
          frame False {
            n11 = call <userlib>:"String Changed__ogtk.vi"("String"=w25) -> ("Changed"=w24:bool)
          }
          frame True {
          }
        }
        n12 = Equal To 0?(x=w17) -> (x = 0?=w16:bool)
        n13 = Compound Arithmetic op=OR(w15, w16) -> (w14:bool)
        n14 = case shown="False" w14 {
          selector: w14 -> [_ w33]
          tunnel: [w27 w36] -> w23
          tunnel: w22 -> [w27 w35]
          tunnel: w17 -> [_ w31]
          tunnel: [_ 1] -> w21
          tunnel: w18 -> [_ w30]
          frame False {
          }
          frame True {
            w29 = "Divider" ("Property.Unique ID string")
            n15 = Bundle By Name(cluster=T2 {"Class Info"={"Unique ID string"="", "Parent ID string"="", "Class Name (unlocalized)"="", "Class Name (localized)"=""}, "Method Info"={"Unique ID string"="", "Data name"="", "Short name (localized)"="", "Long name (localized)"=""}, "Method Flags"={"IsDeprecated"=FALSE, "IsPrivate"=FALSE, "IsScripting"=FALSE, "IsNotInRun-Time"=FALSE}, "Divider"=FALSE} ("element"), "Method Info.Unique ID string"=w29, "Method Info.Data name"=w29, "Method Info.Short name (localized)"=w29, "Method Info.Long name (localized)"=w29, "Class Info.Unique ID string"=w30, "Divider"=w33) -> (w32:T2)
            n16 = Insert Into Array(array=w35, index=w31, new element=w32) -> (w36:T1)
          }
        }
      }
    }
  }
  "Methods[] Out" <- w2
  n17 = Add Array Elements(numeric array=w4) -> (sum=→"Divider Ct":i32)
